vi "close channel.vi"(8 "error in":errorcluster, 11 "DAQ Config":T1) -> (0 "error out":errorcluster)   [LabVIEW 2017, in "Acquisition.lvlib"]
uses:
  Acquisition.lvlib
  Config chanel.ctl
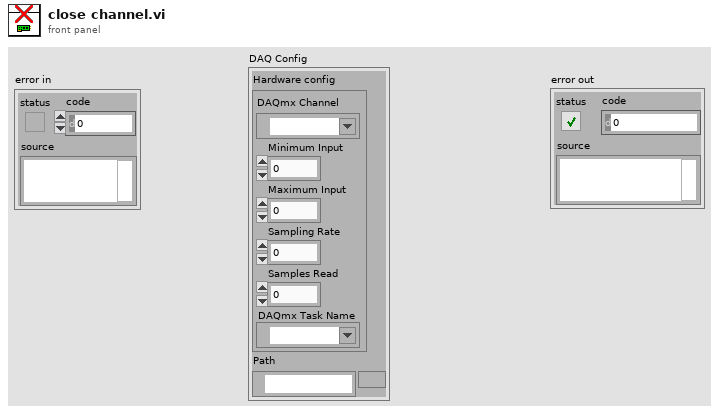
[diagram p1: front panel]
types:
  T1 = typedef "Acquisition.lvlib/Config chanel.ctl" = cluster{"Hardware config":cluster{"DAQmx Channel":tag, "Minimum Input":dbl, "Maximum Input":dbl, "Sampling Rate":dbl, "Samples Read":dbl, "DAQmx Task Name":refnum<k21>}, "Path":path}
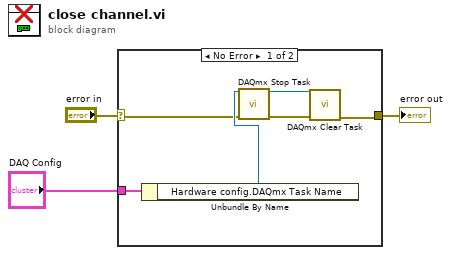
[diagram p0: block diagram]
diagram:
  n1 = case shown="No Error" "error in" {
    selector: "error in" -> [w4 w10]
    tunnel: [w8 w10] -> w2
    tunnel: "DAQ Config" -> [w9 _]
    frame No Error {
      n2 = Unbundle By Name(w9) -> ("Hardware config.DAQmx Task Name"=w5:refnum<k21>)
      n3 = call <vilib>:"DAQmx Stop Task.vi"("task/channels in"=w5, "error in"=w4) -> ("task out"=w6:refnum<k21>, "error out"=w7:errorcluster)  [unwired: 12 in]
      n4 = call <vilib>:"DAQmx Clear Task.vi"("task in"=w6, "error in"=w7) -> ("error out"=w8:errorcluster)  [unwired: 13 in]
    }
    frame Error {
    }
  }
  "error out" <- w2
